vi "Wiimote Get Status Information.vi"(8 "error in":errorcluster, 11 "hWiimoteHandle in":u32 format="%08x") -> (0 "error out":errorcluster, 1 "Battery Level out":u8, 2 "Wiimote LEDs out":T1, 3 "hWiimoteHandle out":u32 format="%08x", 5 "Extension Controller out":bool)   [LabVIEW 2011, in "Wiimote.lvlib"]
uses:
  Wiimote.lvlib
  Wiimote LEDs.ctl
  Wiimote Reporting Mode.ctl
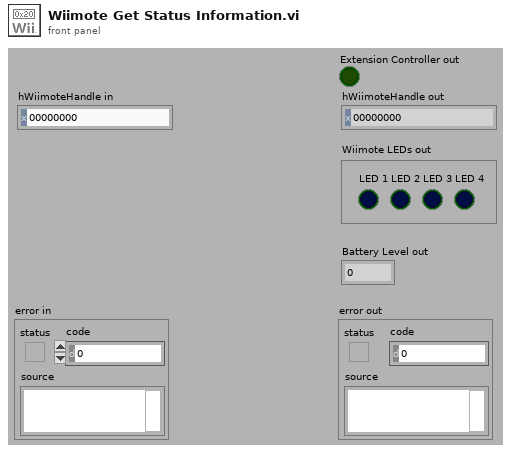
[diagram p1: front panel]
types:
  T1 = typedef "Wiimote.lvlib/Wiimote LEDs.ctl" = cluster{"LED 1":bool, "LED 2":bool, "LED 3":bool, "LED 4":bool}
  T2 = typedef "Wiimote.lvlib/Wiimote Reporting Mode.ctl" = u8
  T3 = cluster{"[0]":bool, "[1]":bool, "[2]":bool, "[3]":bool}
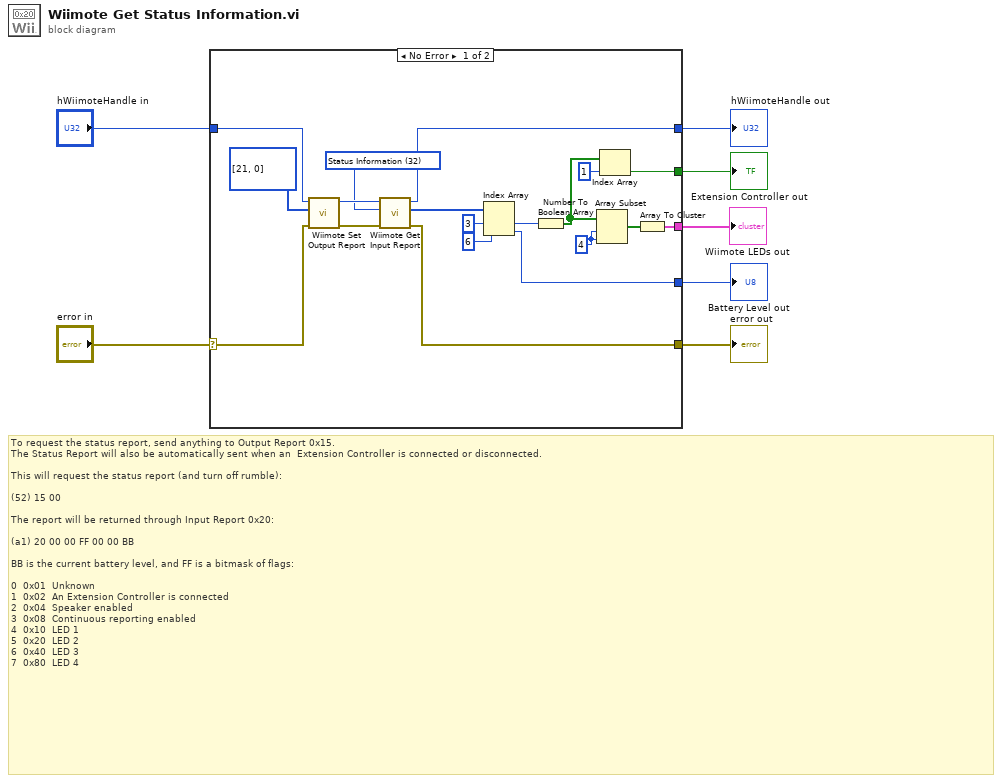
[diagram p0: block diagram]
diagram:
  # "To request the status report, send anything to Output Report 0x15. \nThe Status Report will also be automatically sent when an  Extension Controller is connected or disconnected.\n\nThis will request the status report (and turn off rumble):\n\n(52) 15 00\n\nThe report will be returned through Input Report 0x20:\n\n(a1) 20 00 00 FF 00 00 BB\n\nBB is the current battery level, and FF is a bitmask of flags:\n\n0 \t0x01 \tUnknown\n1 \t0x02 \tAn Extension Controller is connected\n2 \t0x04 \tSpeaker enabled\n3 \t0x08 \tContinuous reporting enabled\n4 \t0x10 \tLED 1\n5 \t0x20 \tLED 2\n6 \t0x40 \tLED 3\n7 \t0x80 \tLED 4"
  n1 = case shown="No Error" "error in" {
    selector: "error in" -> [w24 w28]
    tunnel: [w21 w28] -> w6
    tunnel: "hWiimoteHandle in" -> [w25 w27]
    tunnel: [w20 w27] -> w4
    tunnel: [w15 _] -> w3
    tunnel: [w12 _] -> w2
    tunnel: [w8 _] -> w1
    frame No Error {
      w11 = T2 32 items=["Status Information"=32, "Read Data"=33, "Write Data"=34, "Core Buttons"=48, "Core Buttons and Accelerometer"=49, "Core Buttons with 8 Extension bytes"=50, "Core Buttons and Accelerometer with 12 IR bytes"=51, "Core Buttons with 19 Extension bytes"=52, "Core Buttons and Accelerometer with 16 Extension Bytes"=53, "Core Buttons with 10 IR bytes and 9 Extension Bytes"=54, "Core Buttons and Accelerometer with 10 IR bytes and 6 Extension Bytes"=55] ("bInputReport")
      w14 = 4 ("index")
      n2 = call "Wiimote Set Output Report.vi"("error in"=w24, "pReportBuffer in"=u8[] [21, 0], "hWiimoteHandle in"=w25) -> ("error out"=w22:errorcluster, "hWiimoteHandle out"=w23:u32)  [unwired: 7 in]
      n3 = call "Wiimote Get Input Report.vi"("error in"=w22, "bInputReport"=w11, "hWiimoteHandle in"=w23) -> ("error out"=w21:errorcluster, "pReportBuffer out"=w19:u8[], "hWiimoteHandle out"=w20:u32)  [unwired: 6 in]
      n4 = Index Array(array=w19, index #1=3 ("index"), index #2=6 ("index")) -> (element #1=w17:u8, element #2=w15:u8)
      n5 = Number To Boolean Array(number=w17) -> (Boolean array=w10:bool[])
      n6 = Array Subset(array=w10, index=w14, length=w14) -> (w13:bool[])
      n7 = Index Array(array=w10, index=1) -> (element=w8:bool)
      n8 = Array To Cluster(array=w13) -> (cluster=w12:T3)
    }
    frame Error {
    }
  }
  "error out" <- w6
  "hWiimoteHandle out" <- w4
  "Battery Level out" <- w3
  "Wiimote LEDs out" <- w2
  "Extension Controller out" <- w1
